vi "PFD_get.vi"(0 "PFD_AttitudeControl":cluster{"Roll":sgl, "Pitch":sgl}, 1 "PFD_AltitudeControl":cluster{"Altitude":sgl, "Ground Altitude":sgl}, 2 "PFD_TopControl":T1={"HEARTBEAT"={"type"=enum."MAV_TYPE_GENERIC", "autopilot"=enum."MAV_AUTOPILOT_GENERIC", "custom_mode"=0, "system_status"=enum."MAV_STATE_UNINIT", "mavlink_version"=0, "base_mode"={"CUSTOM_MODE_ENABLED"=FALSE, "TEST_ENABLED"=FALSE, "AUTO_ENABLED"=FALSE, "GUIDED_ENABLED"=FALSE, "STABILIZE_ENABLED"=FALSE, "HIL_ENABLED"=FALSE, "MANUAL_INPUT_ENABLED"=FALSE, "SAFETY_ARMED"=FALSE}, "HEARTBEAT_TIMER"=0, "copter_flight_mode"=enum."Stabilize"}, "Batt Stats"={"Active"=TRUE, "State"=FALSE}, "Sat Stats"={"Active"=TRUE, "State"=FALSE}, "Radio Stats"={"Active"=TRUE, "State"=FALSE}, "Sensor Stats"={"Active"=TRUE, "State"=FALSE}}, 3 "PFD_HeadingControl":sgl format="%#_13g", 4 "PFD_AirSpeedControl":sgl, 5 "PFD_STOP":bool, 6 "PFD_AirSpeedMinMax":cluster{"Max":i16, "Min":i16, "Show":bool}={"Max"=6, "Min"=0, "Show"=TRUE}) -> (10 "PFD_Heading":picture, 12 "PFD_HeadingTop":picture, 13 "PFD_HeadingBack":picture, 14 "PFD_Top":picture, 15 "PFD_Airspeed":picture, 16 "PFD_Attitude":picture, 17 "PFD_Alt":picture, 18 "PFD_AltMid":picture, 19 "PFD_AltShort":picture)   [LabVIEW 2023]
uses:
  PFD_global.vi
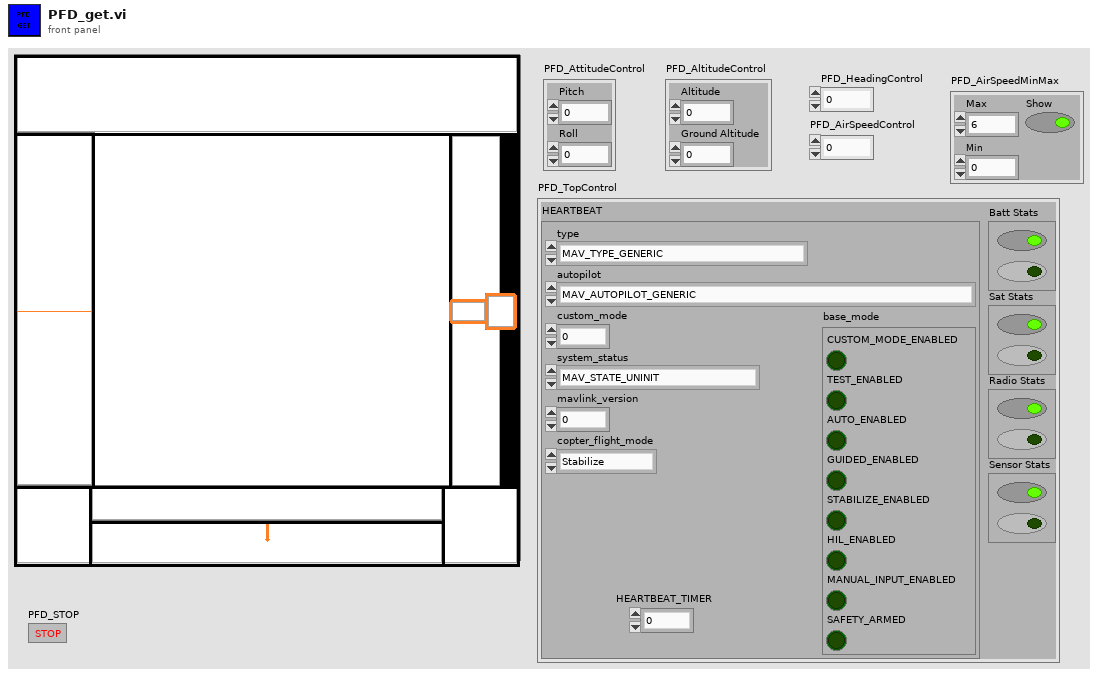
[diagram p1: front panel]
types:
  T1 = cluster{"HEARTBEAT":cluster{"type":enum8{"MAV_TYPE_GENERIC", "MAV_TYPE_FIXED_WING", "MAV_TYPE_QUADROTOR", "MAV_TYPE_COAXIAL", "MAV_TYPE_HELICOPTER", "MAV_TYPE_ANTENNA_TRACKER", "MAV_TYPE_GCS", "MAV_TYPE_AIRSHIP", "MAV_TYPE_FREE_BALLOON", "MAV_TYPE_ROCKET", "MAV_TYPE_GROUND_ROVER", "MAV_TYPE_SURFACE_BOAT", "MAV_TYPE_SUBMARINE", "MAV_TYPE_HEXAROTOR", "MAV_TYPE_OCTOROTOR", "MAV_TYPE_TRICOPTER", "MAV_TYPE_FLAPPING_WING", "MAV_TYPE_KITE", "MAV_TYPE_ONBOARD_CONTROLLER", "MAV_TYPE_VTOL_TAILSITTER_DUOROTOR", "MAV_TYPE_VTOL_TAILSITTER_QUADROTOR", "MAV_TYPE_VTOL_TILTROTOR", "MAV_TYPE_VTOL_FIXEDROTOR", "MAV_TYPE_VTOL_TAILSITTER", "MAV_TYPE_VTOL_TILTWING", "MAV_TYPE_VTOL_RESERVED5", "MAV_TYPE_GIMBAL", "MAV_TYPE_ADSB", "MAV_TYPE_PARAFOIL", "MAV_TYPE_DODECAROTOR", "MAV_TYPE_CAMERA", "MAV_TYPE_CHARGING_STATION", "MAV_TYPE_FLARM", "MAV_TYPE_SERVO", "MAV_TYPE_ODID", "MAV_TYPE_DECAROTOR", "MAV_TYPE_BATTERY", "MAV_TYPE_PARACHUTE", "MAV_TYPE_LOG", "MAV_TYPE_OSD", "MAV_TYPE_IMU", "MAV_TYPE_GPS", "MAV_TYPE_WINCH", "MAV_TYPE_GENERIC_MULTIROTOR", "MAV_TYPE_ILLUMINATOR"}, "autopilot":enum8{"MAV_AUTOPILOT_GENERIC", "MAV_AUTOPILOT_RESERVED", "MAV_AUTOPILOT_SLUGS", "MAV_AUTOPILOT_ARDUPILOTMEGA", "MAV_AUTOPILOT_OPENPILOT", "MAV_AUTOPILOT_GENERIC_WAYPOINTS_ONLY", "MAV_AUTOPILOT_GENERIC_WAYPOINTS_AND_SIMPLE_NAVIGATION_ONLY", "MAV_AUTOPILOT_GENERIC_MISSION_FULL", "MAV_AUTOPILOT_INVALID", "MAV_AUTOPILOT_PPZ", "MAV_AUTOPILOT_UDB", "MAV_AUTOPILOT_FP", "MAV_AUTOPILOT_PX4", "MAV_AUTOPILOT_SMACCMPILOT", "MAV_AUTOPILOT_AUTOQUAD", "MAV_AUTOPILOT_ARMAZILA", "MAV_AUTOPILOT_AEROB", "MAV_AUTOPILOT_ASLUAV", "MAV_AUTOPILOT_SMARTAP", "MAV_AUTOPILOT_AIRRAILS", "MAV_AUTOPILOT_REFLEX"}, "custom_mode":u32, "system_status":enum16{"MAV_STATE_UNINIT", "MAV_STATE_BOOT", "MAV_STATE_CALIBRATING", "MAV_STATE_STANDBY", "MAV_STATE_ACTIVE", "MAV_STATE_CRITICAL", "MAV_STATE_EMERGENCY", "MAV_STATE_POWEROFF", "MAV_STATE_FLIGHT_TERMINATION"}, "mavlink_version":u8, "base_mode":cluster{"CUSTOM_MODE_ENABLED":bool, "TEST_ENABLED":bool, "AUTO_ENABLED":bool, "GUIDED_ENABLED":bool, "STABILIZE_ENABLED":bool, "HIL_ENABLED":bool, "MANUAL_INPUT_ENABLED":bool, "SAFETY_ARMED":bool}, "HEARTBEAT_TIMER":u32, "copter_flight_mode":enum32{"Stabilize", "Acro", "AltHold", "Auto", "Guided", "Loiter", "RTL", "Circle", "--Deprecated-8", "Land", "--Deprecated-10", "Drift", "--Deprecated-12", "Sport", "Flip", "AutoTune", "PosHold", "Brake", "Throw", "Avoid_ADSB", "Guided_NoGPS", "Smart_RTL", "FlowHold", "Follow", "ZigZag", "SystemID", "Heli_Autorotate", "Auto RTL"}}, "Batt Stats":cluster{"Active":bool, "State":bool}, "Sat Stats":cluster{"Active":bool, "State":bool}, "Radio Stats":cluster{"Active":bool, "State":bool}, "Sensor Stats":cluster{"Active":bool, "State":bool}}
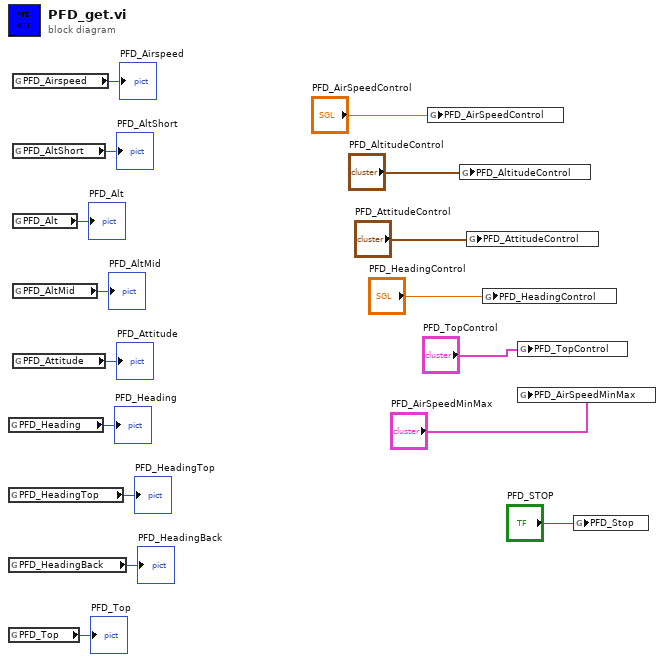
[diagram p0: block diagram]
diagram:
  n1 = global read "PFD_global.vi" "PFD_Heading"() -> (→"PFD_Heading":picture)
  n2 = global read "PFD_global.vi" "PFD_HeadingTop"() -> (→"PFD_HeadingTop":picture)
  n3 = global read "PFD_global.vi" "PFD_HeadingBack"() -> (→"PFD_HeadingBack":picture)
  n4 = global read "PFD_global.vi" "PFD_Top"() -> (→"PFD_Top":picture)
  n5 = global read "PFD_global.vi" "PFD_Airspeed"() -> (→"PFD_Airspeed":picture)
  n6 = global read "PFD_global.vi" "PFD_AltShort"() -> (→"PFD_AltShort":picture)
  n7 = global read "PFD_global.vi" "PFD_Alt"() -> (→"PFD_Alt":picture)
  n8 = global read "PFD_global.vi" "PFD_AltMid"() -> (→"PFD_AltMid":picture)
  n9 = global read "PFD_global.vi" "PFD_Attitude"() -> (→"PFD_Attitude":picture)
  n10 = global write "PFD_global.vi" "PFD_AirSpeedControl"("PFD_AirSpeedControl") -> ()
  n11 = global write "PFD_global.vi" "PFD_AltitudeControl"("PFD_AltitudeControl") -> ()
  n12 = global write "PFD_global.vi" "PFD_AttitudeControl"("PFD_AttitudeControl") -> ()
  n13 = global write "PFD_global.vi" "PFD_HeadingControl"("PFD_HeadingControl") -> ()
  n14 = global write "PFD_global.vi" "PFD_TopControl"("PFD_TopControl") -> ()
  n15 = global write "PFD_global.vi" "PFD_AirSpeedMinMax"("PFD_AirSpeedMinMax") -> ()
  n16 = global write "PFD_global.vi" "PFD_Stop"("PFD_STOP") -> ()
